vi "Motion_Convert Gantry Move Data.vi"(5 "Gantry Move Data":T1 {"Z-Position" format="%_7g"; "Y-Position" format="%_7g"; "X-Position" format="%_7g"; "Gantry Velocity" format="%_7g"; "Gantry Accel/Decel" format="%_7g"}) -> (6 "Gantry Move data":u16[](array[numeric]))   [LabVIEW 2010]
uses:
  Motion_Gantry Position.ctl
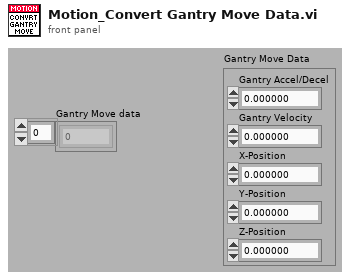
[diagram p1: front panel]
types:
  T1 = typedef "Motion_Gantry Position.ctl" = cluster{"Gantry Accel/Decel":dbl, "Gantry Velocity":dbl, "X-Position":dbl, "Y-Position":dbl, "Z-Position":dbl}
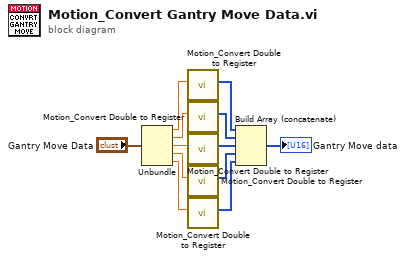
[diagram p0: block diagram]
diagram:
  n1 = Unbundle("Gantry Move Data") -> ("Gantry Accel/Decel"=w5:dbl, "Gantry Velocity"=w4:dbl, "X-Position"=w1:dbl, "Y-Position"=w3:dbl, "Z-Position"=w2:dbl)
  n2 = call "Motion_Convert Double to Register.vi"("Double Value"=w5) -> ("U16 Array"=w12:u16[])  [unwired: 10 in]
  n3 = call "Motion_Convert Double to Register.vi"("Double Value"=w4) -> ("U16 Array"=w11:u16[])  [unwired: 10 in]
  n4 = call "Motion_Convert Double to Register.vi"("Double Value"=w1) -> ("U16 Array"=w10:u16[])  [unwired: 10 in]
  n5 = call "Motion_Convert Double to Register.vi"("Double Value"=w3) -> ("U16 Array"=w9:u16[])  [unwired: 10 in]
  n6 = call "Motion_Convert Double to Register.vi"("Double Value"=w2) -> ("U16 Array"=w8:u16[])  [unwired: 10 in]
  n7 = Build Array (concatenate)(w12, w11, w10, w9, w8) -> (→"Gantry Move data":u16[])
